vi "Stop Core.vi"(10 "final error code":i32, 11 "GUI View in":refnum<class "GUI View.lvclass">) -> (3 "GUI View out":refnum<class "GUI View.lvclass">)   [LabVIEW 2023, in "GUI Views.lvlib" / "GUI View.lvclass"]
doc: "In addition to the following, this method also sends a message to the monitor to notify it that the actor has stopped execution.\n\n(<B>Filename</B>: Actor Framework.lvlib:Actor.lvclass:Stop Core.vi)\n\nDefines what the actor does before it stops. Use the <B>final error code</B> input to determine whether the actor shut down in response to an error.\n\nBy default, this method does nothing. A descendant class may override it to define behavior, such as shutting down any processes the actor initiated in its override of the Actor Core method.\n\nCopyright: MGI\n\nAuthored by Derek Trepanier\nsupport@mooregoodideas.com\nwww.mooregoodideas.com\n\nCopyright (c) 2014, Moore Good Ideas, Inc.\n\nAll rights reserved.\n\nRedistribution and use in source and binary forms, with or without modification, are permitted provided that the following conditions are met:\n\n * Redistributions of source code must retain the above copyright notice, this list of conditions and the following disclaimer.\n * Redistributions in binary form must reproduce the above copyright notice, this list of conditions and the following disclaimer in the documentation and/or other materials provided with the distribution.\n * Neither the name of Moore Good Ideas, Inc. nor the names of its contributors may be used to endorse or promote products derived from this software without specific prior written permission.\n\nTHIS SOFTWARE IS PROVIDED BY THE COPYRIGHT HOLDERS AND CONTRIBUTORS \"AS IS\" AND ANY EXPRESS OR IMPLIED WARRANTIES, INCLUDING, BUT NOT LIMITED TO, THE IMPLIED WARRANTIES OF MERCHANTABILITY AND FITNESS FOR A PARTICULAR PURPOSE ARE DISCLAIMED. IN NO EVENT SHALL THE COPYRIGHT OWNER OR CONTRIBUTORS BE LIABLE FOR ANY DIRECT, INDIRECT, INCIDENTAL, SPECIAL, EXEMPLARY, OR CONSEQUENTIAL DAMAGES (INCLUDING, BUT NOT LIMITED TO, PROCUREMENT OF SUBSTITUTE GOODS OR SERVICES; LOSS OF USE, DATA, OR PROFITS; OR BUSINESS INTERRUPTION) HOWEVER CAUSED AND ON ANY THEORY OF LIABILITY, WHETHER IN CONTRACT, STRICT LIABILITY, OR TORT (INCLUDING NEGLIGENCE OR OTHERWISE) ARISING IN ANY WAY OUT OF THE USE OF THIS SOFTWARE, EVEN IF ADVISED OF THE POSSIBILITY OF SUCH DAMAGE."
uses:
  GUI View.lvclass
  View/View.lvclass
  GUI Container Messages/Remove View with Reply Msg/Remove View with Reply.lvclass
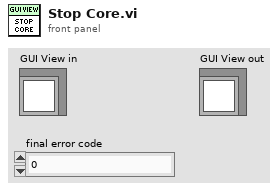
[diagram p1: front panel]
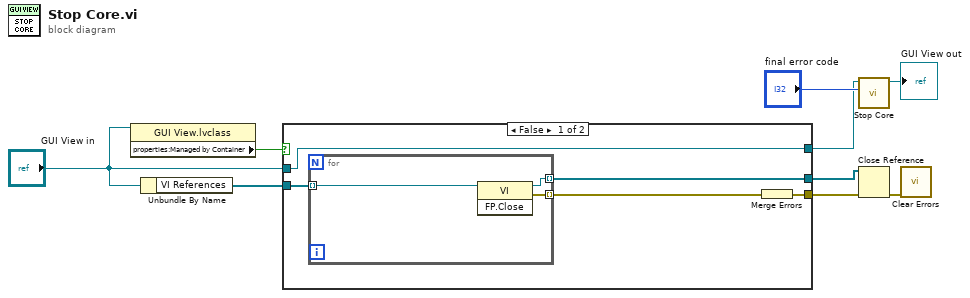
[diagram p0: block diagram]
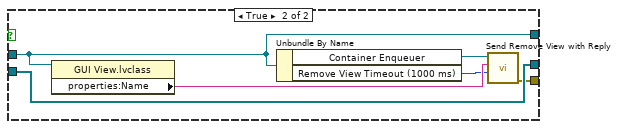
[diagram p2: hidden frame]
diagram:
  n1 = property class="GUI View.lvclass"(reference="GUI View in") -> ("properties:Managed by Container"=w5:bool)  [unwired: 1 in, 2 out]
  n2 = Unbundle By Name("GUI View in") -> ("VI References"=w7:refnum<vi>[])
  n3 = case shown="False" w5 {
    tunnel: w7 -> [w14 w23]
    tunnel: [w13 w23] -> w6
    tunnel: [w11 w22] -> w4
    tunnel: "GUI View in" -> [w10 w18]
    tunnel: [w10 w18] -> w2
    frame False {
      n4 = for {
        tunnel: w14 -> [w17] mode=indexing
        tunnel: [w16] -> w13 mode=indexing
        tunnel: [w15] -> w12 mode=indexing
        n5 = invoke class="VI" method="FP.Close"(reference=w17) -> (reference out=w16:refnum<vi>, error out=w15:errorcluster)  [unwired: 2 in, 1 out]
      }
      n6 = Merge Errors(w12) -> (w11:errorcluster)
    }
    frame True {
      n7 = property class="GUI View.lvclass"(reference=w18) -> ("properties:Name"=w20:string)  [unwired: 1 in, 2 out]
      n8 = Unbundle By Name(w18) -> ("Container Enqueuer"=w21:refnum<class "Message Enqueuer.lvclass">, "Remove View Timeout (1000 ms)"=w19:i32)
      n9 = call "Send Remove View with Reply.vi"("timeout in ms (-1)"=w19, "View"=w20, "Message Enqueuer in"=w21) -> ("error out"=w22:errorcluster)  [unwired: 7 in, 1 out]
    }
  }
  n10 = call-parent "Stop Core.vi"("final error code"="final error code", "Actor in"=w2) -> ("Actor out"=→"GUI View out":refnum<class "GUI View.lvclass">)  [unwired: 9 in]
  n11 = Close Reference(reference=w6, error in (no error)=w4) -> (error out=w1:errorcluster)
  n12 = call <vilib>:"Clear Errors.vi"("error in (no error)"=w1) -> ()  [unwired: 5 in, 2 out]
